vi "Package Error Info.vi"(8 "error in":errorcluster, 11 "String in":string) -> (0 "packed error info out":string=": general error code 0, ", 3 "error status":bool)   [LabVIEW 2017]
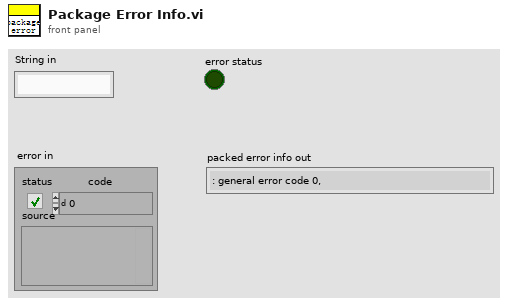
[diagram p1: front panel]
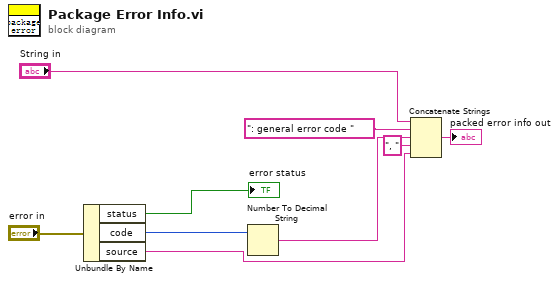
[diagram p0: block diagram]
diagram:
  n1 = Unbundle By Name("error in") -> ("status"=→"error status":bool, "code"=w7:i32, "source"=w2:string)
  n2 = Number To Decimal String(number=w7) -> (decimal integer string=w4:string)  [unwired: 1 in]
  n3 = Concatenate Strings("String in", ": general error code " ("string"), w4, ", " ("string"), w2) -> (→"packed error info out":string)
